vi "Perform Action.vi"(8 "error in":errorcluster, 10 "Input":variant, 11 "AI DAQmx Cont CFG in":refnum<class "AI DAQmx Cont CFG.lvclass">) -> (0 "error out":errorcluster, 2 "Output":variant, 3 "AI DAQmx Cont CFG out":refnum<class "AI DAQmx Cont CFG.lvclass">)   [LabVIEW 2023, in "AI DAQmx Cont CFG.lvclass"]
uses:
  AI DAQmx Cont CFG.lvclass
  AI DAQmx Cont CFG.lvclass/AI DAQmx Cont CFG.ctl
  DAQmx/DAQmx Base CFG/DAQmx Base CFG.lvclass/DAQmx Base CFG.ctl
  Configuration/Configuration Semaphore/CFG Semaphore.lvclass/CFG Semaphore.ctl
  <vilib>/DAQmx/read.llb/DAQmx Read (Analog 2D DBL NChan NSamp).vi
  <vilib>/DAQmx/miscellaneous.llb/DAQmx Fill In Error Info.vi
  DAQmx/BufferLastReadingsDBL/BufferLastReadings DBL.lvclass
  DAQmx/DAQmx Base CFG/DAQmx Base CFG.lvclass
  <resource>/objmgr/daqmx.rc
  Configuration/Configuration Semaphore/CFG Semaphore.lvclass
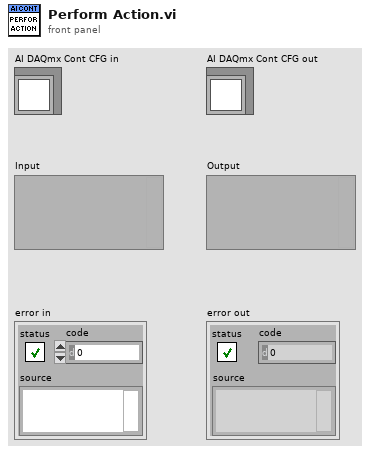
[diagram p1: front panel]
types:
  T1 = typedef "Semaphore RefNum" = refnum<k1>
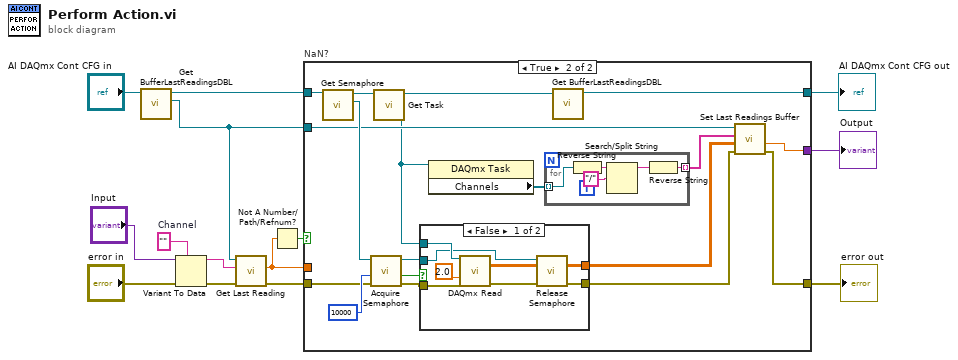
[diagram p0: block diagram]
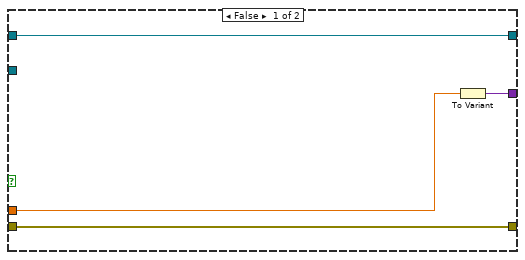
[diagram p2: hidden frame]
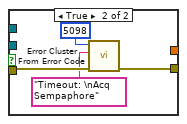
[diagram p3: hidden frame]
diagram:
  w12 = ""  # Channel
  n1 = call "Get BufferLastReadingsDBL.vi"("AI DAQmx Cont CFG in"="AI DAQmx Cont CFG in") -> ("BufferLastReadings DBL"=w4:refnum<class "BufferLastReadings DBL.lvclass">, "AI DAQmx Cont CFG out"=w8:refnum<class "AI DAQmx Cont CFG.lvclass">)  [unwired: 9 in]
  n2 = Variant To Data(error in="error in", type=w12, Variant="Input") -> (data=w7:string, error out=w6:errorcluster)
  n3 = call-dynamic "Get Last Reading.vi"("error in"=w6, "Channel"=w7, "BufferLastReadingsDBL in"=w4) -> ("error out"=w1:errorcluster, "Reading"=w2:dbl)  [unwired: 6 in, 1 out]
  n4 = Not A Number/Path/Refnum?(number/path/refnum=w2) -> (NaN/Path/Refnum?=w5:bool)
  n5 = case "NaN?" shown="True" w5 {
    tunnel: [w15 w22] -> w10
    tunnel: [w16 w32] -> w9
    tunnel: w8 -> [w16 w30]
    tunnel: w4 -> [_ w31]
    tunnel: [w17 w21] -> w3
    tunnel: w2 -> [w18 _]
    tunnel: w1 -> [w15 w20]
    frame False {
      n6 = To Variant(anything=w18) -> (Variant=w17:variant)
    }
    frame True {
      n7 = call "Get Semaphore.vi"("CFG Base in"=w30) -> ("Semaphore"=w36:T1, "CFG Base out"=w29:refnum<class "AI DAQmx Cont CFG.lvclass">)  [unwired: 9 in]
      n8 = call <vilib>:"Acquire Semaphore.vi"("error in (no error)"=w20, "ms timeout (-1)"=10000, "semaphore"=w36) -> ("error out"=w34:errorcluster, "timed out"=w35:bool, "semaphore out"=w19:T1)  [unwired: 2 in]
      n9 = call "Get Task.vi"("DAQmx Base CFG in"=w29) -> ("Task"=w27:refnum<k21>, "DAQmx Base CFG out"=w28:refnum<class "AI DAQmx Cont CFG.lvclass">)  [unwired: 9 in]
      n10 = case shown="False" w35 {
        tunnel: [w43 w52] -> w23
        tunnel: w34 -> [w47 w51]
        tunnel: w27 -> [w45 _]
        tunnel: [w44 _] -> w24
        tunnel: w19 -> [w42 _]
        frame False {
          n11 = call-poly <vilib>:"DAQmx Read.vi"("task/channels in"=w45, "timeout"=2.0, "error in"=w47) -> ("data"=w44:dbl[][], "error out"=w48:errorcluster)  [unwired: 10 in, 1 out]
          n12 = call <vilib>:"Release Semaphore.vi"("error in (no error)"=w48, "semaphore"=w42) -> ("error out"=w43:errorcluster)  [unwired: 4 in, 1 out]
        }
        frame True {
          n13 = call <vilib>:"Error Cluster From Error Code.vi"("error in (no error)"=w51, "error message (\"\")"="Timeout: \nAcq Sempaphore" ("error message (\"\")"), "error code (0)"=5098) -> ("error out"=w52:errorcluster)  [unwired: 6 in]
        }
      }
      n14 = property class="DAQmx Task"(reference=w27) -> ("Channels"=w26:refnum<k21>[])  [unwired: 1 in, 2 out]
      n15 = for {
        tunnel: w26 -> [w37] mode=indexing
        tunnel: [w38] -> w25 mode=indexing
        n16 = Reverse String(1:w37) -> (0:w40:string)
        n17 = Search/Split String(string=w40, search string/char (-)="/") -> (substring before match=w39:string)  [unwired: 1 in, 2 out]
        n18 = Reverse String(1:w39) -> (0:w38:string)
      }
      n19 = call "Get BufferLastReadingsDBL.vi"("AI DAQmx Cont CFG in"=w28) -> ("AI DAQmx Cont CFG out"=w32:refnum<class "AI DAQmx Cont CFG.lvclass">)  [unwired: 9 in, 1 out]
      n20 = call-dynamic "Set Last Readings Buffer.vi"("error in"=w23, "Readings"=w24, "Channel Idents"=w25, "BufferLastReadingsDBL in"=w31) -> ("error out"=w22:errorcluster, "Reading"=w21:dbl)  [unwired: 5 in, 1 out]
    }
  }
  "error out" <- w10
  "AI DAQmx Cont CFG out" <- w9
  "Output" <- w3
